vi "SV Append Waveform (1 Ch) (DBL).vi"(7 "reset (F)":bool, 8 "error in (no error)":errorcluster, 10 "maximum length [s] (-1 = unlimited)":dbl=-1.0, 11 "waveform data in":waveform(dbl)) -> (0 "error out":errorcluster, 3 "appended waveform data":waveform(dbl))   [LabVIEW 2017]
doc: "Use this VI to buffer data by appending input data to previously buffered data. Set the <B>maximum length</B> to set the buffered array size. The VI functions like a FIFO (First In, First Out) buffer, meaning that the oldest data is overwritten as new elements are added to the buffer. Wire data to the <B>data in</B> input to determine the polymorphic instance to use or manually select the instance."
uses:
  <vilib>/addons/_NISVFA/_Shared subVIs/Common/svc_Get Waveform Subset (Index).vi
  <vilib>/addons/_NISVFA/_Shared subVIs/Common/svc_Check for Waveform Parameter Continuity (no state).vi
  <vilib>/addons/_NISVFA/_Shared subVIs/Common/svc_Get Array Subset (Index).vi
  <vilib>/addons/_NISVFA/_Shared subVIs/Common/svc_Get SV Channel Info.vi
  <vilib>/addons/_NISVFA/_Shared subVIs/Common/svc_Coerce Index and Length.vi
  <vilib>/addons/_NISVFA/_Shared subVIs/Common/svc_Conditional Merge Error.vi
  <vilib>/addons/_NISVFA/_Shared subVIs/Common/svc_Engineering Units to Unit Label.vi
  <vilib>/addons/_NISVFA/_Shared subVIs/Common/svc_Unit Label to Engineering Units.vi
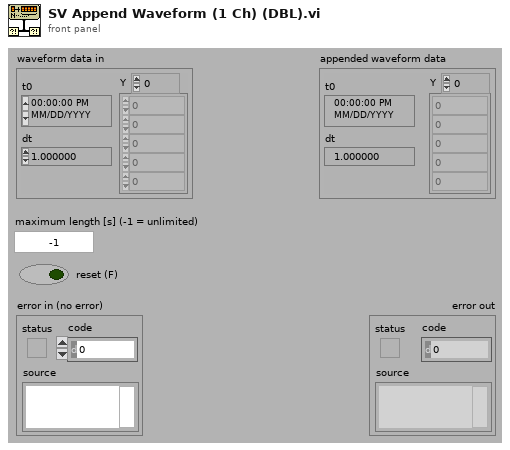
[diagram p1: front panel]
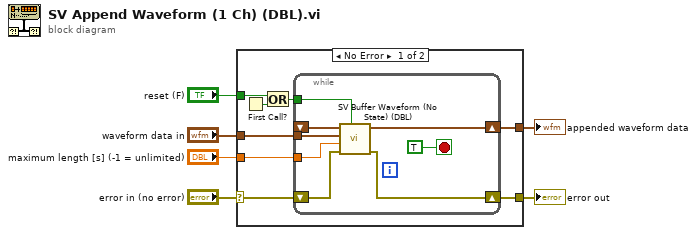
[diagram p0: block diagram]
diagram:
  n1 = case shown="No Error" "error in (no error)" {
    selector: "error in (no error)" -> [w7 w23]
    tunnel: "reset (F)" -> [w14 _]
    tunnel: [w12 w24] -> w5
    tunnel: "maximum length [s] (-1 = unlimited)" -> [w11 _]
    tunnel: "waveform data in" -> [w10 w24]
    tunnel: [w8 w23] -> w2
    frame No Error {
      n2 = First Call?() -> (First Call?: T/F=w9:bool)
      n3 = Or(x=w14, y=w9) -> (x .or. y?=w13:bool)
      n4 = while {
        tunnel: w10 -> [w20]
        shift-right: [w22] -> w12
        shift-left: _ -> [w21]
        tunnel: w11 -> [w17]
        tunnel: w13 -> [w19]
        shift-right: [w15] -> w8
        shift-left: w7 -> [w16]
        stop <- TRUE stop-if-true
        n5 = call <vilib>:"SV Buffer Waveform (No State) (DBL).vi"("clear buffer (False)"=w19, "error in (no error)"=w16, "buffer length [s] (-1 = unlimited)"=w17, "waveform"=w20, "buffer in"=w21) -> ("error out"=w15:errorcluster, "buffer out"=w22:waveform(dbl))  [unwired: 5 in]
      }
    }
    frame Error {
    }
  }
  "appended waveform data" <- w5
  "error out" <- w2
